vi "Create Channel Task Manual.vi"(8 "error in":errorcluster, 9 "Waveform Generation":T1(array[cluster]), 10 "SQL query":string="SELECT max(MaximumVoltage),max(MinimumVoltage), max(TerminalConfiguration),max(SampleRate) FROM ltt.daq_configuration \nWhere ChannelType='Waveform_Output' and Enabled=1;", 11 "NI Waveform Output in":refnum<class "NI Waveform Output.lvclass">) -> (0 "error out":errorcluster, 3 "NI Waveform Output out":refnum<class "NI Waveform Output.lvclass">)   [LabVIEW 2023, in "HardwareAbstractionLayer_LVOOP.lvlib" / "NI Waveform Output.lvclass"]
doc: "This VI Analog Output Physical Channel Based DAQmx Create Channel"
uses:
  NI Waveform Output.lvclass
  NI Waveform Output.lvclass/NI Waveform Output.ctl
  <vilib>/DAQmx/create/channels.llb/DAQmx Create Channel (AO-Voltage-Basic).vi
  <vilib>/DAQmx/configure/timing.llb/DAQmx Timing (Sample Clock).vi
  Database/Database.lvclass
panel:
  # "SELECT max(MaximumVoltage),max(MinimumVoltage), max(TerminalConfiguration),max(SampleRate) FROM ltt.daq_configuration \nWhere ChannelType='Waveform_Output' and Enabled=1;"
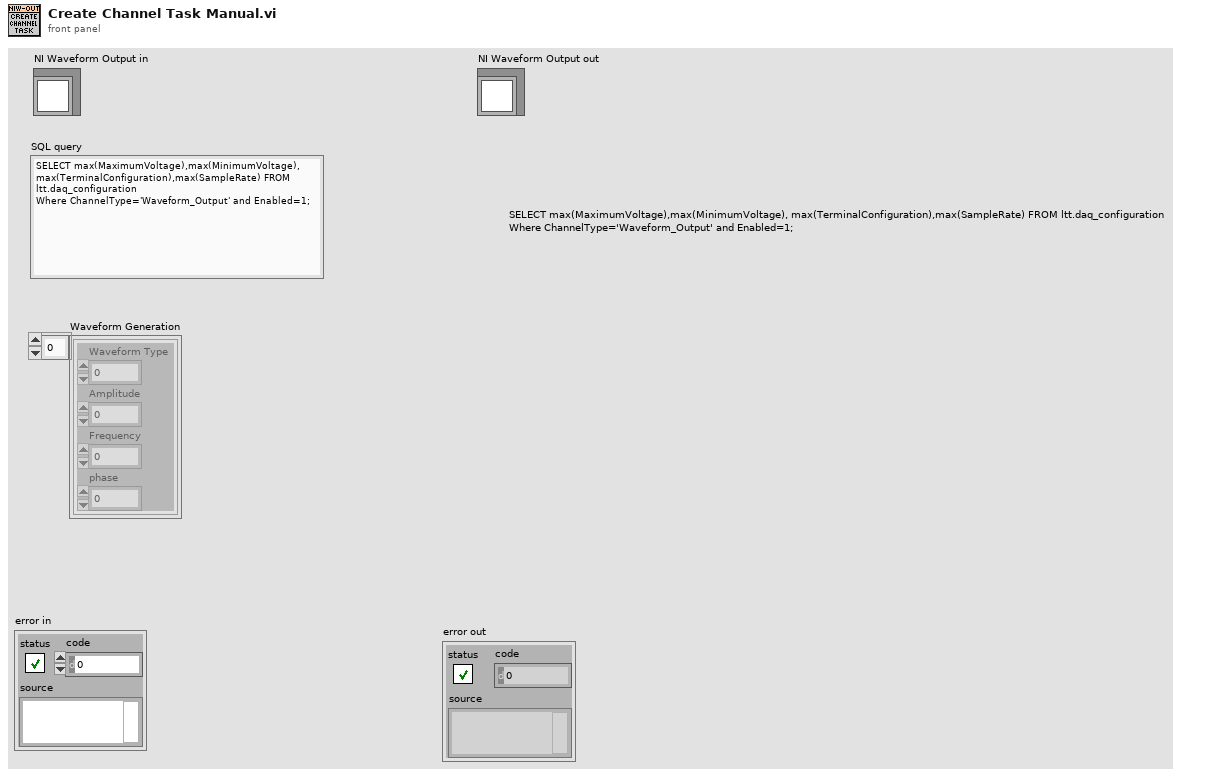
[diagram p1: front panel]
types:
  T1 = cluster{"Waveform Type":u16, "Amplitude":dbl, "Frequency":dbl, "phase":dbl}[]
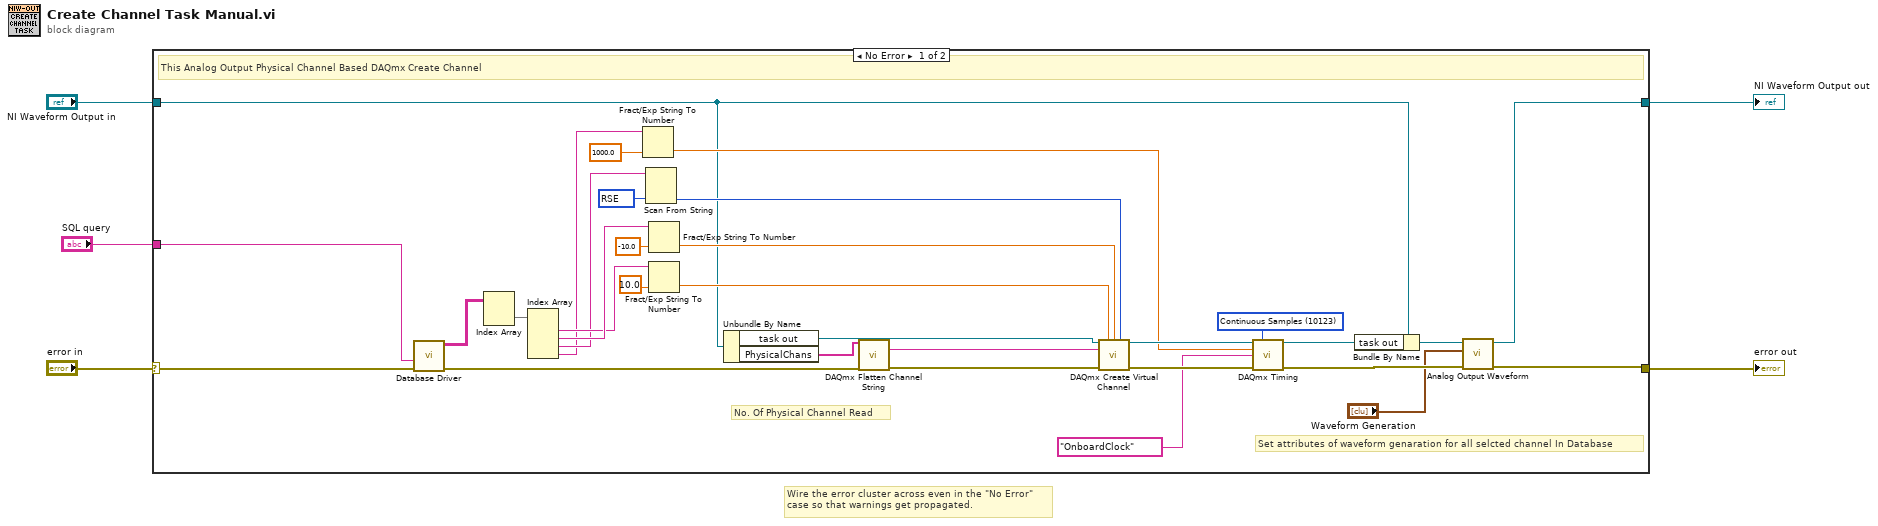
[diagram p0: block diagram]
diagram:
  # "Wire the error cluster across even in the \"No Error\"\ncase so that warnings get propagated."
  n1 = case shown="No Error" "error in" {
    selector: "error in" -> [w16 w39]
    tunnel: [w8 w39] -> w4
    tunnel: [w7 w38] -> w2
    tunnel: "NI Waveform Output in" -> [w12 w38]
    tunnel: "SQL query" -> [w11 _]
    frame No Error {
      w18 = 10123 items=["Finite Samples"=10178, "Continuous Samples"=10123, "Hardware Timed Single Point"=12522] ("sample mode")
      w34 = 10083 items=["Default"=-1, "RSE"=10083, "NRSE"=10078, "Differential"=10106, "Pseudodifferential"=12529] ("input terminal configuration")
      # "Set attributes of waveform genaration for all selcted channel In Database"
      # "No. Of Physical Channel Read"
      # "This Analog Output Physical Channel Based DAQmx Create Channel"
      n2 = call "Database Driver.vi"("error in"=w16, "SQL query"=w11) -> ("error out"=w14:errorcluster, "data"=w15:string[][])  [unwired: 6 in, 2 out]
      n3 = Index Array(array=w15) -> (element=w35:string[])  [unwired: 2 in]
      n4 = Index Array(array=w35) -> (element #1=w36:string, element #2=w37:string, element #3=w28:string, element #4=w20:string)  [unwired: 4 in]
      n5 = Fract/Exp String To Number(string=w20, default (0 dbl)=1000.0 ("rate")) -> (number=w19:dbl)  [unwired: 2 in, 1 out]
      n6 = Scan From String(input string=w28, default 1=w34) -> (output 1=w29:i32)  [unwired: 3 in, 3 out]
      n7 = Fract/Exp String To Number(string=w37, default (0 dbl)=-10.0 ("maximum value")) -> (number=w30:dbl)  [unwired: 2 in, 1 out]
      n8 = Fract/Exp String To Number(string=w36, default (0 dbl)=10.0 ("maximum value")) -> (number=w31:dbl)  [unwired: 2 in, 1 out]
      n9 = Unbundle By Name(w12) -> ("task out"=w24:refnum<k21>, "PhysicalChans"=w26:tag[])
      n10 = call <vilib>:"DAQmx Flatten Channel String.vi"("names in"=w26, "error in"=w14) -> ("names out"=w25:string, "error out"=w27:errorcluster)  [unwired: 12 in]
      n11 = call-poly <vilib>:"DAQmx Create Virtual Channel.vi"("task in"=w24, "maximum value"=w31, "minimum value"=w30, "output terminal configuration"=w29, "physical channels"=w25, "error in"=w27) -> ("task out"=w22:refnum<k21>, "error out"=w23:errorcluster)  [unwired: 8 in]
      n12 = call-poly <vilib>:"DAQmx Timing.vi"("task/channels in"=w22, "sample mode"=w18, "rate"=w19, "source"=tag "OnboardClock", "error in"=w23) -> ("task out"=w17:refnum<k21>, "error out"=w9:errorcluster)  [unwired: 9 in]
      n13 = Bundle By Name(cluster=w12, "task out"=w17) -> (w10:refnum<class "NI Waveform Output.lvclass">)
      n14 = call-dynamic "Analog Output Waveform.vi"("error in (no error)"=w9, "Waveform Generation"="Waveform Generation", "NI Waveform Output in"=w10) -> ("error out"=w8:errorcluster, "NI Waveform Output out"=w7:refnum<class "NI Waveform Output.lvclass">)  [unwired: 7 in]
    }
    frame Error {
    }
  }
  "error out" <- w4
  "NI Waveform Output out" <- w2
